vi "ControlChanged.vi"(4 "Changed Names in (empty)":string[](array[string]), 5 "timeout in ms (1000ms)":i32=1000, 6 "Prefix (\"\")":string, 7 "ControlToCommand":map{refnum<vi>, string[]}(c390), 8 "IO Queue":refnum<queue>, 9 "NewVal":variant, 10 "OldVal":variant, 11 "CtlRef":refnum<vi>) -> (0 "Changed Names out":string[](array[string]))   [LabVIEW 2021, in "TextControlledInstrum.lvlib"]
uses:
  TextControlledInstrum.lvlib
  IOQueuePacket.ctl
  <vilib>/regexp/Match Regular Expression.xnode
  <vilib>/Utility/Data Type/NI_Data Type.lvlib
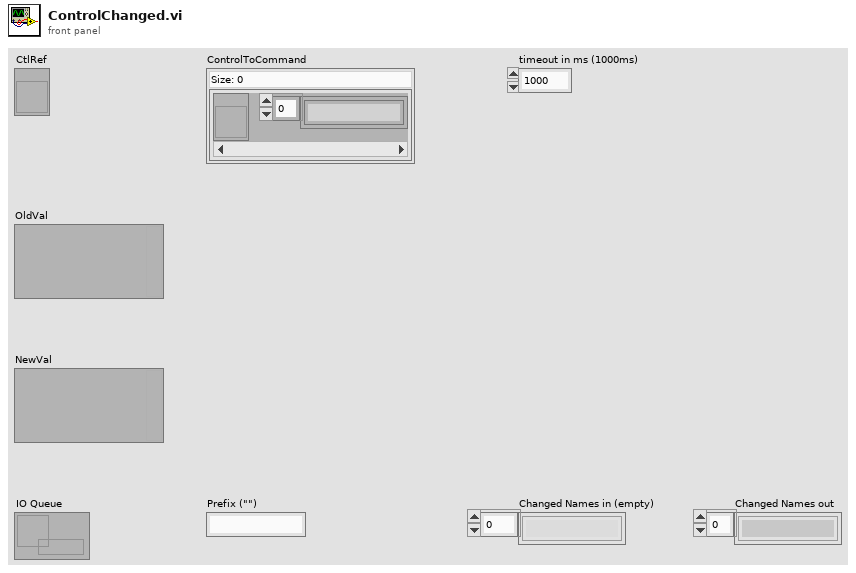
[diagram p1: front panel]
types:
  T1 = typedef "NI_Data Type.lvlib/Data Type.ctl" = enum8{"Invalid Type", "Void", "I8", "I16", "I32", "I64", "U8", "U16", "U32", "U64", "Single Float", "Double Float", "Extended Float", "Single Complex", "Double Complex", "Extended Complex", "Enum U8", "Enum U16", "Enum U32", "Enum U64", "Single Float With Unit", "Double Float With Unit", "Extended Float With Unit", "Single Complex with Unit", "Double Complex with Unit", "Extended Complex with Unit", "Boolean", "String", "Path", "Picture", "Tag", "Array", "Cluster", "Variant", "LV Variant", "Waveform", "Timestamp", "Digital Waveform", "Digital Data", "ExpressData", "Refnum", "External Data", "VI", "Poly VI", "LabVIEW Class Instance", "Fixed Point", "Set Collection", "Map Collection"}
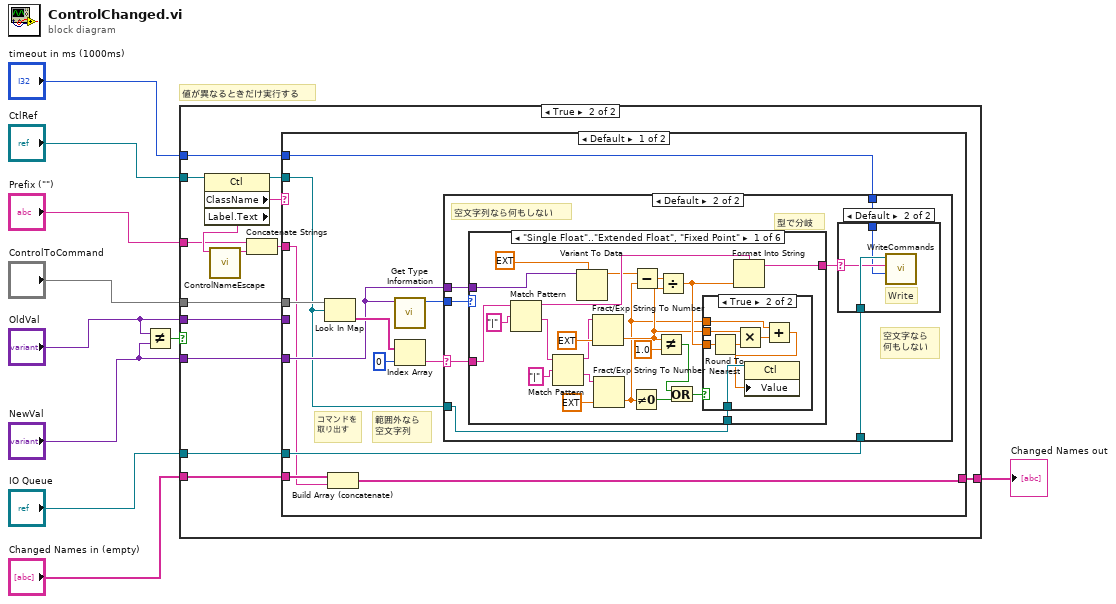
[diagram p0: block diagram]
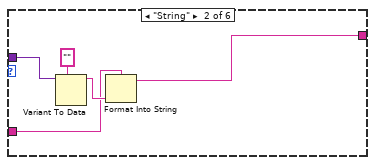
[diagram p6: hidden frame]
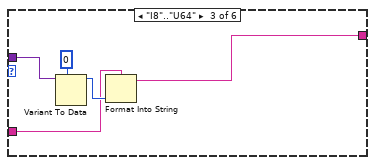
[diagram p7: hidden frame]
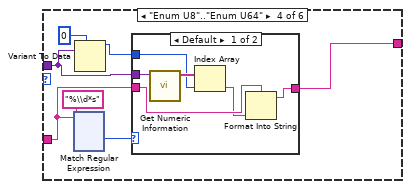
[diagram p8: hidden frame]
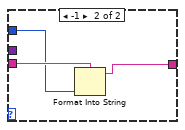
[diagram p9: hidden frame]
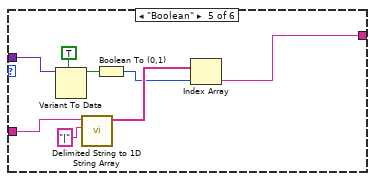
[diagram p10: hidden frame]
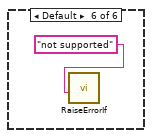
[diagram p11: hidden frame]
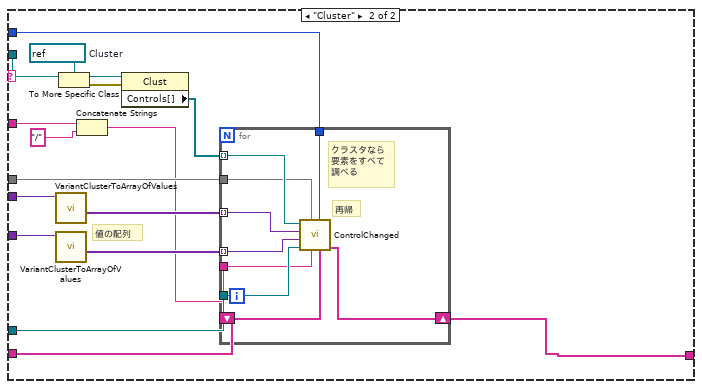
[diagram p12: hidden frame]
diagram:
  # "値が異なるときだけ実行する"
  n1 = Not Equal?(x="OldVal", y="NewVal") -> (x != y?=w6:bool)
  n2 = case shown="True" w6 {
    tunnel: "IO Queue" -> [_ w24]
    tunnel: "CtlRef" -> [_ w22]
    tunnel: "ControlToCommand" -> [_ w21]
    tunnel: "OldVal" -> [_ w20]
    tunnel: "NewVal" -> [_ w19]
    tunnel: "timeout in ms (1000ms)" -> [_ w18]
    tunnel: "Prefix (\"\")" -> [_ w15]
    tunnel: "Changed Names in (empty)" -> [w11 w13]
    tunnel: [w11 w12] -> w1
    frame False {
    }
    frame True {
      n3 = property class="Ctl"(reference=w22) -> (reference out=w23:refnum<vi>, "ClassName"=w25:string, "Label.Text"=w16:string)  [unwired: 1 in, 1 out]
      n4 = call "ControlNameEscape.vi"("label"=w16) -> ("escaped string"=w17:string)  [unwired: 10 in]
      n5 = Concatenate Strings(w15, w17) -> (w14:string)
      n6 = case shown="Default" w25 {
        tunnel: w20 -> [_ w243]
        tunnel: w19 -> [w32 w242]
        tunnel: w24 -> [w31 w241]
        tunnel: w23 -> [w26 w240]
        tunnel: w21 -> [w37 w235]
        tunnel: w18 -> [w30 w234]
        tunnel: w14 -> [w28 w233]
        tunnel: w13 -> [w29 w230]
        tunnel: [w27 w229] -> w12
        frame Default {
          # "範囲外なら\n空文字列"
          # "コマンドを\n取り出す"
          n7 = Look In Map(map=w37, key=w26) -> (value=w33:string[])  [unwired: 1 in, 1 out]
          n8 = Build Array (concatenate)(w29, w28) -> (w27:string[])
          n9 = call <vilib>:"Get Type Information.vi"("variant"=w32) -> ("type"=w36:T1)  [unwired: 6 in, 4 out]
          n10 = Index Array(array=w33, index=0 ("index (row)")) -> (element=w34:string)
          n11 = case shown="Default" w34 {
            selector: w34 -> [_ w41]
            tunnel: w36 -> [_ w44]
            tunnel: w32 -> [_ w43]
            tunnel: w31 -> [_ w42]
            tunnel: w30 -> [_ w39]
            tunnel: w26 -> [_ w38]
            frame "" {
            }
            frame Default {
              # "空文字なら\n何もしない"
              # "型で分岐"
              # "空文字列なら何もしない"
              n12 = case shown="\"Single Float\"..\"Extended Float\", \"Fixed Point\"" w44 {
                tunnel: w43 -> [w69 w81 w86 w89 w225 _]
                tunnel: w41 -> [w65 w77 w82 w87 w227 _]
                tunnel: [w67 w79 w84 w90 w220 _] -> w40
                tunnel: w38 -> [w48 _ _ _ _ _]
                frame "Single Float".."Extended Float", "Fixed Point" {
                  n13 = Match Pattern(string=w65, regular expression="|") -> (before substring=w64:string, after substring=w61:string)  [unwired: 1 in, 2 out]
                  n14 = Match Pattern(string=w61, regular expression="|") -> (before substring=w59:string, after substring=w58:string)  [unwired: 1 in, 2 out]
                  n15 = Variant To Data(type=ext 0.0, Variant=w69) -> (data=w57:ext)  [unwired: 1 in, 1 out]
                  n16 = Fract/Exp String To Number(string=w59, default (0 dbl)=ext 1.0 ("default (0 DBL)")) -> (number=w50:ext)  [unwired: 2 in, 1 out]
                  n17 = Fract/Exp String To Number(string=w58, default (0 dbl)=ext 0.0 ("default (0 DBL)")) -> (number=w49:ext)  [unwired: 2 in, 1 out]
                  n18 = Not Equal To 0?(x=w49) -> (x != 0?=w54:bool)
                  n19 = Subtract(x=w57, y=w49) -> (x-y=w56:ext)
                  n20 = Not Equal?(x=w50, y=1.0) -> (x != y?=w53:bool)
                  n21 = Divide(x=w56, y=w50) -> (x/y=w51:ext)
                  n22 = Or(x=w53, y=w54) -> (x .or. y?=w52:bool)
                  n23 = case shown="True" w52 {
                    tunnel: w51 -> [_ w76]
                    tunnel: w50 -> [_ w74]
                    tunnel: w49 -> [_ w72]
                    tunnel: w48 -> [_ w71]
                    frame False {
                    }
                    frame True {
                      n24 = Round To Nearest(number=w76) -> (nearest integer value=w75:ext)
                      n25 = Multiply(x=w74, y=w75) -> (x*y=w73:ext)
                      n26 = Add(x=w72, y=w73) -> (x+y=w70:ext)
                      n27 = property class="Ctl"(reference=w71, "Value"=w70) -> ()  [unwired: 1 in, 2 out]
                    }
                  }
                  n28 = Format Into String(format string=w64, w51) -> (resulting string=w67:string)  [unwired: 2 in, 1 out]
                }
                frame "String" {
                  n29 = Variant To Data(type="", Variant=w81) -> (data=w80:string)  [unwired: 1 in, 1 out]
                  n30 = Format Into String(format string=w77, w80) -> (resulting string=w79:string)  [unwired: 2 in, 1 out]
                }
                frame "I8".."U64" {
                  n31 = Variant To Data(type=i64 0, Variant=w86) -> (data=w85:i64)  [unwired: 1 in, 1 out]
                  n32 = Format Into String(format string=w82, w85) -> (resulting string=w84:string)  [unwired: 2 in, 1 out]
                }
                frame "Enum U8".."Enum U64" {
                  n33 = xnode "Match Regular Expression"("input string"=w87, "regular expression"="%\\d*s" ("input string")) -> ("offset past match"=w93:i32)  [unwired: 4 in, 4 out]
                  n34 = Variant To Data(type=0, Variant=w89) -> (data=w91:i32)  [unwired: 1 in, 1 out]
                  n35 = case shown="Default" w93 {
                    tunnel: w87 -> [w96 w102]
                    tunnel: w91 -> [w97 w101]
                    tunnel: [w94 w100] -> w90
                    tunnel: w89 -> [w99 _]
                    frame Default {
                      n36 = call <vilib>:"Get Numeric Information.vi"("variant"=w99) -> ("enum names"=w98:string[])  [unwired: 7 in, 3 out]
                      n37 = Index Array(array=w98, index=w97) -> (element=w95:string)
                      n38 = Format Into String(format string=w96, w95) -> (resulting string=w94:string)  [unwired: 2 in, 1 out]
                    }
                    frame -1 {
                      n39 = Format Into String(format string=w102, w101) -> (resulting string=w100:string)  [unwired: 2 in, 1 out]
                    }
                  }
                }
                frame "Boolean" {
                  n40 = Variant To Data(type=TRUE, Variant=w225) -> (data=w223:bool)  [unwired: 1 in, 1 out]
                  n41 = call <vilib>:"Delimited String to 1D String Array.vi"("delimiter"="|", "delimited string"=w227) -> ("string array"=w222:string[])  [unwired: 9 in]
                  n42 = Boolean To (0,1)(Boolean=w223) -> (0, 1=w221:i16)
                  n43 = Index Array(array=w222, index=w221) -> (element=w220:string)
                }
                frame Default {
                  n44 = call "RaiseErrorIf.vi"("error message"="not supported" ("error source (\" \")")) -> ()  [unwired: 10 in, 1 out]
                }
              }
              n45 = case shown="Default" w40 {
                selector: w40 -> [_ w46]
                tunnel: w42 -> [_ w47]
                tunnel: w39 -> [_ w45]
                frame "" {
                }
                frame Default {
                  # "Write"
                  n46 = call "WriteCommands.vi"("timeout in ms (100)"=w45, "Multi-line String"=w46, "IO Queue"=w47) -> ()  [unwired: 7 in, 2 out]
                }
              }
            }
          }
        }
        frame "Cluster" {
          w239 = refnum<vi> refnum  # Cluster
          # "値の配列"
          n47 = call "VariantClusterToArrayOfValues.vi"("Cluster Variant"=w243) -> ("Values"=w245:variant[])  [unwired: 8 in, 2 out]
          n48 = call "VariantClusterToArrayOfValues.vi"("Cluster Variant"=w242) -> ("Values"=w244:variant[])  [unwired: 8 in, 2 out]
          n49 = To More Specific Class(target class=w239, reference=w240) -> (specific class reference=w238:refnum<vi>, error out=w237:errorcluster)  [unwired: 1 in]
          n50 = Concatenate Strings(w233, "/" ("string")) -> (w231:string)
          n51 = property class="Clust"(reference=w238, error in=w237) -> ("Controls[]"=w236:refnum<vi>[])  [unwired: 2 out]
          n52 = for {
            tunnel: w245 -> [w253] mode=indexing
            tunnel: w244 -> [w252] mode=indexing
            tunnel: w241 -> [w251]
            tunnel: w234 -> [w250]
            tunnel: w236 -> [w254] mode=indexing
            tunnel: w235 -> [w249]
            tunnel: w231 -> [w248]
            shift-right: [w246] -> w229
            shift-left: w230 -> [w247]
            # "クラスタなら\n要素をすべて\n調べる"
            # "再帰"
            n53 = call "ControlChanged.vi"("Changed Names in (empty)"=w247, "timeout in ms (1000ms)"=w250, "Prefix (\"\")"=w248, "ControlToCommand"=w249, "IO Queue"=w251, "NewVal"=w252, "OldVal"=w253, "CtlRef"=w254) -> ("Changed Names out"=w246:string[])  [unwired: 3 in]
          }
        }
      }
    }
  }
  "Changed Names out" <- w1
